vi "Excit_Format_Wfm_Name.vi"(7 "Excit Number":i32, 8 "error in":errorcluster, 11 "EXCIT Waveforms Inputs":T1={"Excit Form"=enum."Swift", "Swift Factor"=0.5, "Chirp Apodisation"=3.5, "Duration"=800.0, "Intensity"=100.0, "Start Frequency"=250.0, "End Frequency"=1000.0, "Intensity 2"=100.0, "Start Frequency 2"=250.0, "End Frequency 2"=350.0, "Sampling Frequency"=5.0} caption="EXCIT Inputs" {"End Frequency 2" min=1.0 max=10000.0; "Start Frequency 2" min=1.0 max=10000.0; "Intensity 2" min=1.0 max=100.0; "Chirp Apodisation" min=1.0 max=5.0 step=0.1; "Swift Factor" min=0.1 max=3.0 step=0.1; "Sampling Frequency" min=1.0 max=100.0 step=1.0; "Duration" min=1.0 max=1000000.0 step=1.0; "End Frequency" min=1.0 max=10000.0; "Start Frequency" min=1.0 max=10000.0 step=0.1 format="%#.6g"; "Intensity" min=1.0 max=100.0}) -> (0 "error out":errorcluster caption="sortie d'erreur", 3 "Waveform Name":string)   [LabVIEW 2017]
doc: "From a start and end value, generates an adiabatic waveform signal of 2000 values (double).\nWrites this waveform into a binary file, in a big-endian format.\nDisplays the written data and the FFT of the signal.\nDefault Path for the generated file is D:\\PIRENEA\\EXCIT_WFMS\n\nAvailable Waveforms : Sinus, Swift, Chirp, Ramp (Up or Down), DoubleRamp (Up-Down or Down-Up)"
uses:
  controls/EXCIT_Waveform_Inputs.ctl
  controls/EXCIT_Form_Selector.ctl
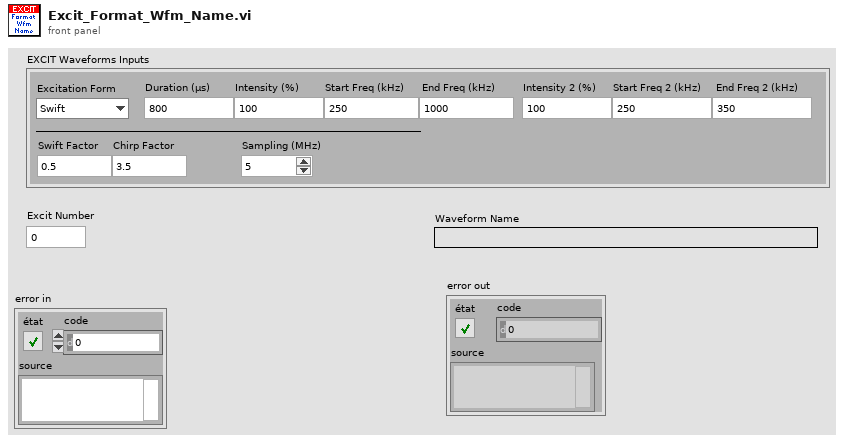
[diagram p1: front panel]
types:
  T1 = typedef "EXCIT_Waveform_Inputs.ctl" = cluster{"Excit Form":T2, "Swift Factor":dbl, "Chirp Apodisation":dbl, "Duration":dbl, "Intensity":dbl, "Start Frequency":dbl, "End Frequency":dbl, "Intensity 2":dbl, "Start Frequency 2":dbl, "End Frequency 2":dbl, "Sampling Frequency":dbl}
  T2 = typedef "EXCIT_Form_Selector.ctl" = enum16{"Swift", "TwoSwift", "Chirp", "Sinus", "Ramp"}
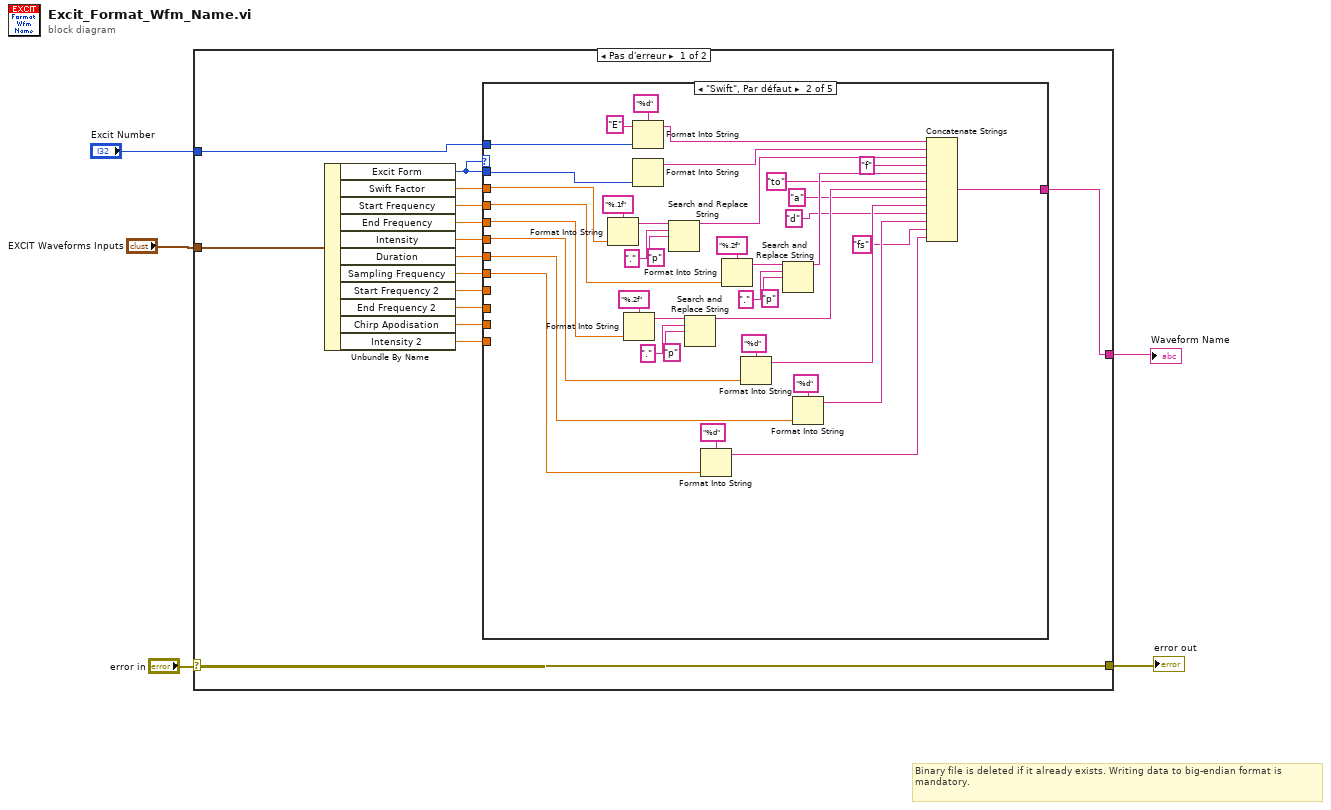
[diagram p0: block diagram]
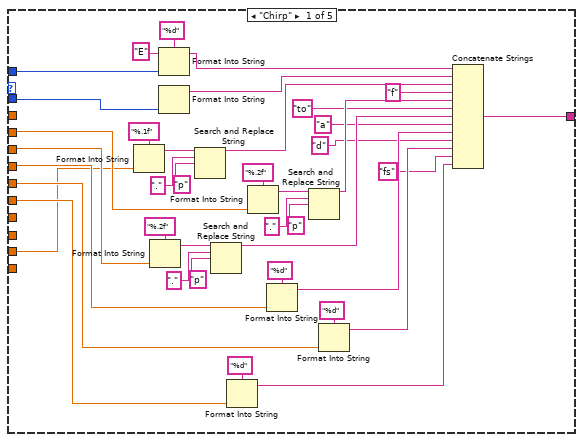
[diagram p2: hidden frame]
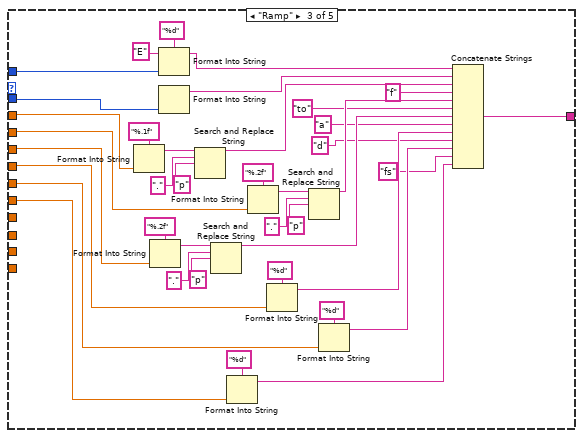
[diagram p3: hidden frame]
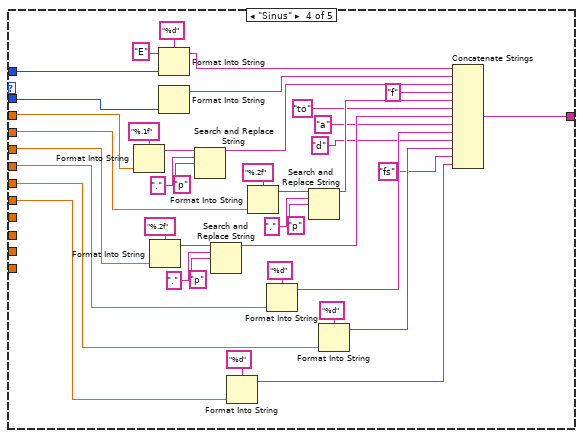
[diagram p4: hidden frame]
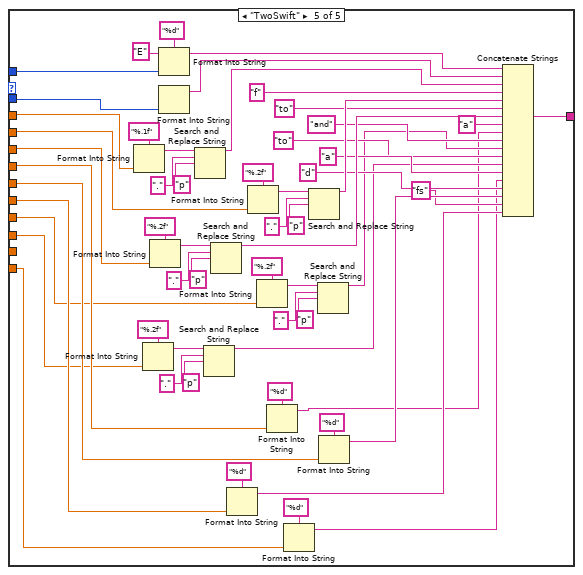
[diagram p5: hidden frame]
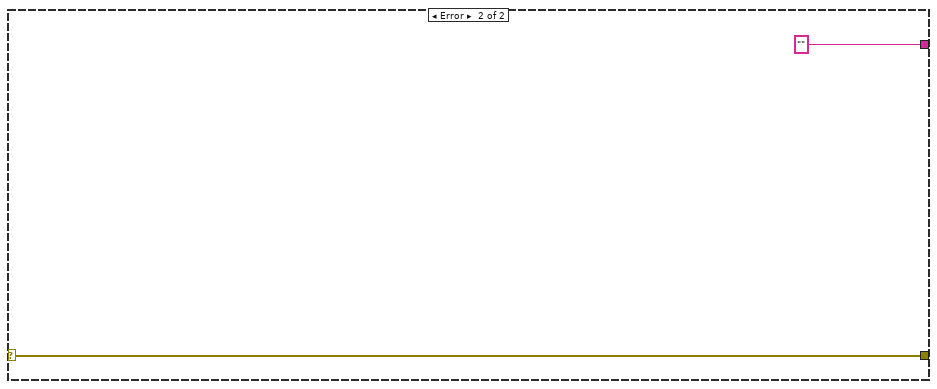
[diagram p6: hidden frame]
diagram:
  # "Binary file is deleted if it already exists. Writing data to big-endian format is mandatory."
  n1 = case shown="Pas d'erreur" "error in" {
    selector: "error in" -> [w12 w235]
    tunnel: [w12 w235] -> w5
    tunnel: [w11 ""] -> w3
    tunnel: "EXCIT Waveforms Inputs" -> [w19 _]
    tunnel: "Excit Number" -> [w20 _]
    frame No Error {
      n2 = Unbundle By Name(w19) -> ("Excit Form"=w10:T2, "Swift Factor"=w18:dbl, "Start Frequency"=w17:dbl, "End Frequency"=w16:dbl, "Intensity"=w15:dbl, "Duration"=w14:dbl, "Sampling Frequency"=w13:dbl, "Start Frequency 2"=w8:dbl, "End Frequency 2"=w7:dbl, "Chirp Apodisation"=w9:dbl, "Intensity 2"=w6:dbl)
      n3 = case shown="\"Swift\", Par défaut" w10 {
        tunnel: w10 -> [w59 w98 w137 w176 w233]
        tunnel: w20 -> [w58 w97 w136 w175 w232]
        tunnel: w18 -> [_ w96 w135 w174 w231]
        tunnel: w17 -> [w57 w95 w134 w173 w230]
        tunnel: w16 -> [w56 w94 w133 w172 w229]
        tunnel: w15 -> [w55 w93 w132 w171 w228]
        tunnel: w14 -> [w54 w92 w131 w170 w227]
        tunnel: w13 -> [w53 w91 w130 w169 w199]
        tunnel: [w23 w61 w100 w139 w201] -> w11
        tunnel: w9 -> [w21 _ _ _ _]
        tunnel: w8 -> [_ _ _ _ w192]
        tunnel: w7 -> [_ _ _ _ w186]
        tunnel: w6 -> [_ _ _ _ w178]
        frame "Chirp" {
          n4 = Format Into String(format string="%.1f" ("chaîne de format"), w21) -> (resulting string=w45:string)  [unwired: 2 in, 1 out]
          n5 = Format Into String(format string="%.2f" ("chaîne de format"), w56) -> (resulting string=w34:string)  [unwired: 2 in, 1 out]
          n6 = Format Into String(format string="%d" ("chaîne de format"), initial string="E" ("chaîne initiale"), w58) -> (resulting string=w50:string)  [unwired: 1 in, 1 out]
          n7 = Format Into String(w59) -> (resulting string=w49:string)  [unwired: 3 in, 1 out]
          n8 = Search and Replace String(input string=w45, search string="." ("chaîne recherchée"), replace string="p" ("chaîne de remplacement (\"\")")) -> (result string=w44:string)  [unwired: 5 in, 3 out]
          n9 = Search and Replace String(input string=w34, search string="." ("chaîne recherchée"), replace string="p" ("chaîne de remplacement (\"\")")) -> (result string=w33:string)  [unwired: 5 in, 3 out]
          n10 = Format Into String(format string="%d" ("chaîne de format"), w53) -> (resulting string=w24:string)  [unwired: 2 in, 1 out]
          n11 = Format Into String(format string="%.2f" ("chaîne de format"), w57) -> (resulting string=w43:string)  [unwired: 2 in, 1 out]
          n12 = Format Into String(format string="%d" ("chaîne de format"), w55) -> (resulting string=w31:string)  [unwired: 2 in, 1 out]
          n13 = Search and Replace String(input string=w43, search string="." ("chaîne recherchée"), replace string="p" ("chaîne de remplacement (\"\")")) -> (result string=w39:string)  [unwired: 5 in, 3 out]
          n14 = Format Into String(format string="%d" ("chaîne de format"), w54) -> (resulting string=w29:string)  [unwired: 2 in, 1 out]
          n15 = Concatenate Strings(w50, w49, w44, "f" ("chaîne"), w39, "to" ("chaîne"), w33, "a" ("chaîne"), w31, "d" ("chaîne"), w29, "fs" ("chaîne"), w24) -> (w23:string)
        }
        frame "Swift", Default {
          n16 = Format Into String(format string="%.1f" ("chaîne de format"), w96) -> (resulting string=w83:string)  [unwired: 2 in, 1 out]
          n17 = Format Into String(format string="%.2f" ("chaîne de format"), w94) -> (resulting string=w72:string)  [unwired: 2 in, 1 out]
          n18 = Format Into String(format string="%d" ("chaîne de format"), initial string="E" ("chaîne initiale"), w97) -> (resulting string=w88:string)  [unwired: 1 in, 1 out]
          n19 = Format Into String(w98) -> (resulting string=w87:string)  [unwired: 3 in, 1 out]
          n20 = Search and Replace String(input string=w83, search string="." ("chaîne recherchée"), replace string="p" ("chaîne de remplacement (\"\")")) -> (result string=w82:string)  [unwired: 5 in, 3 out]
          n21 = Search and Replace String(input string=w72, search string="." ("chaîne recherchée"), replace string="p" ("chaîne de remplacement (\"\")")) -> (result string=w71:string)  [unwired: 5 in, 3 out]
          n22 = Format Into String(format string="%d" ("chaîne de format"), w91) -> (resulting string=w62:string)  [unwired: 2 in, 1 out]
          n23 = Format Into String(format string="%.2f" ("chaîne de format"), w95) -> (resulting string=w81:string)  [unwired: 2 in, 1 out]
          n24 = Format Into String(format string="%d" ("chaîne de format"), w93) -> (resulting string=w69:string)  [unwired: 2 in, 1 out]
          n25 = Search and Replace String(input string=w81, search string="." ("chaîne recherchée"), replace string="p" ("chaîne de remplacement (\"\")")) -> (result string=w77:string)  [unwired: 5 in, 3 out]
          n26 = Format Into String(format string="%d" ("chaîne de format"), w92) -> (resulting string=w67:string)  [unwired: 2 in, 1 out]
          n27 = Concatenate Strings(w88, w87, w82, "f" ("chaîne"), w77, "to" ("chaîne"), w71, "a" ("chaîne"), w69, "d" ("chaîne"), w67, "fs" ("chaîne"), w62) -> (w61:string)
        }
        frame "Ramp" {
          n28 = Format Into String(format string="%.1f" ("chaîne de format"), w135) -> (resulting string=w122:string)  [unwired: 2 in, 1 out]
          n29 = Format Into String(format string="%.2f" ("chaîne de format"), w133) -> (resulting string=w111:string)  [unwired: 2 in, 1 out]
          n30 = Format Into String(format string="%d" ("chaîne de format"), initial string="E" ("chaîne initiale"), w136) -> (resulting string=w127:string)  [unwired: 1 in, 1 out]
          n31 = Format Into String(w137) -> (resulting string=w126:string)  [unwired: 3 in, 1 out]
          n32 = Search and Replace String(input string=w122, search string="." ("chaîne recherchée"), replace string="p" ("chaîne de remplacement (\"\")")) -> (result string=w121:string)  [unwired: 5 in, 3 out]
          n33 = Search and Replace String(input string=w111, search string="." ("chaîne recherchée"), replace string="p" ("chaîne de remplacement (\"\")")) -> (result string=w110:string)  [unwired: 5 in, 3 out]
          n34 = Format Into String(format string="%d" ("chaîne de format"), w130) -> (resulting string=w101:string)  [unwired: 2 in, 1 out]
          n35 = Format Into String(format string="%.2f" ("chaîne de format"), w134) -> (resulting string=w120:string)  [unwired: 2 in, 1 out]
          n36 = Format Into String(format string="%d" ("chaîne de format"), w132) -> (resulting string=w108:string)  [unwired: 2 in, 1 out]
          n37 = Search and Replace String(input string=w120, search string="." ("chaîne recherchée"), replace string="p" ("chaîne de remplacement (\"\")")) -> (result string=w116:string)  [unwired: 5 in, 3 out]
          n38 = Format Into String(format string="%d" ("chaîne de format"), w131) -> (resulting string=w106:string)  [unwired: 2 in, 1 out]
          n39 = Concatenate Strings(w127, w126, w121, "f" ("chaîne"), w116, "to" ("chaîne"), w110, "a" ("chaîne"), w108, "d" ("chaîne"), w106, "fs" ("chaîne"), w101) -> (w100:string)
        }
        frame "Sinus" {
          n40 = Format Into String(format string="%.1f" ("chaîne de format"), w174) -> (resulting string=w161:string)  [unwired: 2 in, 1 out]
          n41 = Format Into String(format string="%.2f" ("chaîne de format"), w172) -> (resulting string=w150:string)  [unwired: 2 in, 1 out]
          n42 = Format Into String(format string="%d" ("chaîne de format"), initial string="E" ("chaîne initiale"), w175) -> (resulting string=w166:string)  [unwired: 1 in, 1 out]
          n43 = Format Into String(w176) -> (resulting string=w165:string)  [unwired: 3 in, 1 out]
          n44 = Search and Replace String(input string=w161, search string="." ("chaîne recherchée"), replace string="p" ("chaîne de remplacement (\"\")")) -> (result string=w160:string)  [unwired: 5 in, 3 out]
          n45 = Search and Replace String(input string=w150, search string="." ("chaîne recherchée"), replace string="p" ("chaîne de remplacement (\"\")")) -> (result string=w149:string)  [unwired: 5 in, 3 out]
          n46 = Format Into String(format string="%d" ("chaîne de format"), w169) -> (resulting string=w140:string)  [unwired: 2 in, 1 out]
          n47 = Format Into String(format string="%.2f" ("chaîne de format"), w173) -> (resulting string=w159:string)  [unwired: 2 in, 1 out]
          n48 = Format Into String(format string="%d" ("chaîne de format"), w171) -> (resulting string=w147:string)  [unwired: 2 in, 1 out]
          n49 = Search and Replace String(input string=w159, search string="." ("chaîne recherchée"), replace string="p" ("chaîne de remplacement (\"\")")) -> (result string=w155:string)  [unwired: 5 in, 3 out]
          n50 = Format Into String(format string="%d" ("chaîne de format"), w170) -> (resulting string=w145:string)  [unwired: 2 in, 1 out]
          n51 = Concatenate Strings(w166, w165, w160, "f" ("chaîne"), w155, "to" ("chaîne"), w149, "a" ("chaîne"), w147, "d" ("chaîne"), w145, "fs" ("chaîne"), w140) -> (w139:string)
        }
        frame "TwoSwift" {
          n52 = Format Into String(format string="%.1f" ("chaîne de format"), w231) -> (resulting string=w221:string)  [unwired: 2 in, 1 out]
          n53 = Format Into String(format string="%.2f" ("chaîne de format"), w186) -> (resulting string=w187:string)  [unwired: 2 in, 1 out]
          n54 = Format Into String(format string="%.2f" ("chaîne de format"), w229) -> (resulting string=w211:string)  [unwired: 2 in, 1 out]
          n55 = Format Into String(format string="%d" ("chaîne de format"), initial string="E" ("chaîne initiale"), w232) -> (resulting string=w184:string)  [unwired: 1 in, 1 out]
          n56 = Format Into String(w233) -> (resulting string=w183:string)  [unwired: 3 in, 1 out]
          n57 = Search and Replace String(input string=w221, search string="." ("chaîne recherchée"), replace string="p" ("chaîne de remplacement (\"\")")) -> (result string=w182:string)  [unwired: 5 in, 3 out]
          n58 = Search and Replace String(input string=w187, search string="." ("chaîne recherchée"), replace string="p" ("chaîne de remplacement (\"\")")) -> (result string=w185:string)  [unwired: 5 in, 3 out]
          n59 = Search and Replace String(input string=w211, search string="." ("chaîne recherchée"), replace string="p" ("chaîne de remplacement (\"\")")) -> (result string=w210:string)  [unwired: 5 in, 3 out]
          n60 = Format Into String(format string="%d" ("chaîne de format"), w199) -> (resulting string=w202:string)  [unwired: 2 in, 1 out]
          n61 = Format Into String(format string="%.2f" ("chaîne de format"), w230) -> (resulting string=w220:string)  [unwired: 2 in, 1 out]
          n62 = Format Into String(format string="%.2f" ("chaîne de format"), w192) -> (resulting string=w196:string)  [unwired: 2 in, 1 out]
          n63 = Format Into String(format string="%d" ("chaîne de format"), w228) -> (resulting string=w180:string)  [unwired: 2 in, 1 out]
          n64 = Format Into String(format string="%d" ("chaîne de format"), w178) -> (resulting string=w177:string)  [unwired: 2 in, 1 out]
          n65 = Search and Replace String(input string=w220, search string="." ("chaîne recherchée"), replace string="p" ("chaîne de remplacement (\"\")")) -> (result string=w216:string)  [unwired: 5 in, 3 out]
          n66 = Search and Replace String(input string=w196, search string="." ("chaîne recherchée"), replace string="p" ("chaîne de remplacement (\"\")")) -> (result string=w191:string)  [unwired: 5 in, 3 out]
          n67 = Format Into String(format string="%d" ("chaîne de format"), w227) -> (resulting string=w207:string)  [unwired: 2 in, 1 out]
          n68 = Concatenate Strings(w184, w183, w182, "f" ("chaîne"), w216, "to" ("chaîne"), w210, "a" ("chaîne"), w180, "and" ("chaîne"), w191, "to" ("chaîne"), w185, "a" ("chaîne"), w177, "d" ("chaîne"), w207, "fs" ("chaîne"), w202) -> (w201:string)
        }
      }
    }
    frame Error {
    }
  }
  "error out" <- w5
  "Waveform Name" <- w3
